vi "Run Server.vi"(8 "error in (no error)":errorcluster, 11 "Stop OOB Server UE":refnum<user-event>) -> (0 "error out":errorcluster)   [LabVIEW 2025, in "ExamplePluginOOBService_server.lvlib"]
uses:
  ExamplePluginOOBService_server.lvlib
  <vilib>/gRPC/LabVIEW gRPC Servicer/Servicer/Servicer.lvclass
  <vilib>/gRPC/LabVIEW gRPC Servicer/ServiceBase/ServiceBase.lvclass
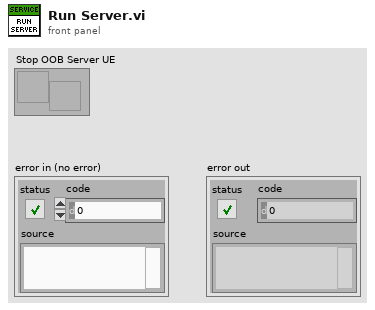
[diagram p1: front panel]
types:
  T1 = enum32{"Invalid", "Standard", "Closed", "Hidden", "Minimized", "Maximized"}
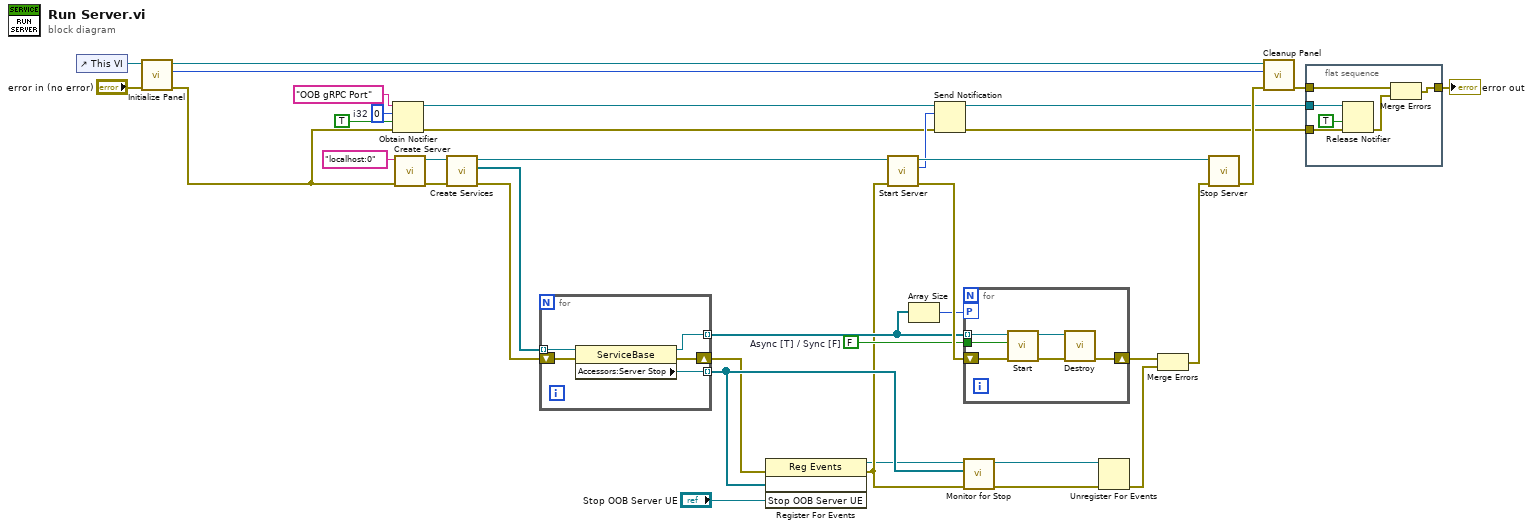
[diagram p0: block diagram]
diagram:
  w10 = 0  # i32
  w32 = FALSE  # Async [T] / Sync [F]
  n1 = control-ref of="This VI"() -> (w21:refnum<vi>)
  n2 = call "Initialize Panel.vi"("error in (no error)"="error in (no error)", "vi reference in"=w21) -> ("error out"=w11:errorcluster, "initial window state"=w19:T1, "vi reference out"=w20:refnum<vi>)  [unwired: 7 in]
  n3 = Obtain Notifier(name (unnamed)="OOB gRPC Port", notification data type=w10, create if not found? (T)=TRUE, error in (no error)=w11) -> (notifier out=w8:refnum<notifier>, error out=w2:errorcluster)  [unwired: 1 out]
  n4 = call <vilib>:"Create Server.vi"("error in"=w11, "Server Address"="localhost:0") -> ("error out"=w17:errorcluster, "gRPC server out"=w35:refnum<class "Servicer.lvclass">)  [unwired: 8 in]
  n5 = call "Create Services.vi"("error in (no error)"=w17, "gRPC server in"=w35) -> ("error out"=w16:errorcluster, "gRPC services out"=w15:refnum<class "ServiceBase.lvclass">[], "gRPC server out"=w34:refnum<class "Servicer.lvclass">)  [unwired: 7 in]
  n6 = for {
    tunnel: [w41] -> w29 mode=indexing
    shift-right: [w40] -> w28
    shift-left: w16 -> [w38]
    tunnel: [w42] -> w30 mode=indexing
    tunnel: w15 -> [w39] mode=indexing
    n7 = property class="ServiceBase"(reference=w39, error in=w38) -> (reference out=w42:refnum<class "ServiceBase.lvclass">, error out=w40:errorcluster, "Accessors:Server Stop"=w41:refnum<user-event>)
  }
  n8 = register-events(error in=w28, w29, "Stop OOB Server UE") -> (reference out=w12:refnum<event-registration>, error out=w27:errorcluster)  [unwired: 1 in]
  n9 = call <vilib>:"Start Server.vi"("error in"=w27, "gRPC server in"=w34) -> ("error out"=w33:errorcluster, "Listening Port"=w7:i32, "gRPC server out"=w37:refnum<class "Servicer.lvclass">)  [unwired: 7 in]
  n10 = Array Size(array=w30) -> (size(s)=w31:i32)
  n11 = Send Notification(notification=w7, notifier=w8, error in (no error)=w2) -> (notifier out=w6:refnum<notifier>, error out=w3:errorcluster)
  n12 = for {
    tunnel: w30 -> [w46] mode=indexing
    tunnel: w32 -> [w44]
    workers-P: w31 -> [_]
    shift-right: [w43] -> w26
    shift-left: w33 -> [w45]
    n13 = call-dynamic "Start.vi"("error in"=w45, "ASync [T]"=w44, "gRPC service in"=w46) -> ("error out"=w47:errorcluster, "gRPC service out"=w48:refnum<class "ServiceBase.lvclass">)  [unwired: 7 in]
    n14 = call-dynamic "Destroy.vi"("error in"=w47, "gRPC service in"=w48) -> ("error out"=w43:errorcluster)  [unwired: 8 in, 1 out]
  }
  n15 = call "Monitor for Stop.vi"("error in (no error)"=w27, "service stop events"=w29, "Event Registration Refnum in"=w12) -> ("error out"=w22:errorcluster, "Event Registration Refnum out"=w24:refnum<event-registration>)  [unwired: 7 in]
  n16 = Unregister For Events(event registration refnum=w24, error in=w22) -> (error out=w23:errorcluster)
  n17 = Merge Errors(w26, w23) -> (w25:errorcluster)
  n18 = call <vilib>:"Stop Server.vi"("error in"=w25, "gRPC server in"=w37) -> ("error out"=w18:errorcluster)  [unwired: 9 in]
  n19 = call "Cleanup Panel.vi"("error in (no error)"=w18, "initial window state"=w19, "vi reference in"=w20) -> ("error out"=w5:errorcluster)  [unwired: 7 in, 1 out]
  n20 = flat-sequence {
    tunnel: w6 -> [w54]
    tunnel: w5 -> [w52]
    tunnel: [w51] -> w4
    tunnel: w3 -> [w49]
    frame #0 {
      n21 = Release Notifier(notifier=w54, force destroy? (F)=TRUE, error in (no error)=w49) -> (error out=w50:errorcluster)  [unwired: 2 out]
      n22 = Merge Errors(w52, w50) -> (w51:errorcluster)
    }
  }
  "error out" <- w4
